vi "Source and Measure Current in DMM.vi"() -> ()   [LabVIEW 2021]
uses:
  <instrlib>/niDCPower/nidcpower.llb/niDCPower Source Mode.ctl
  <instrlib>/niDCPower/nidcpower.llb/niDCPower Wait For Event - Event.ctl
  <instrlib>/niDCPower/nidcpower.llb/niDCPower Output Function.ctl
  <instrlib>/niDMM/nidmm.llb/niDMM Function.ctl
  <instrlib>/niDMM/nidmm.llb/niDMM Configure Measurement Digits.vi
  <instrlib>/Agilent 3446X Series/Public/Data/Read (Single Point).vi
  <instrlib>/Agilent N6700 Series/Agilent N6700 Series.lvlib
  <instrlib>/Agilent 3446X Series/Agilent 3446X Series.lvlib
panel:
  in  "Agilent SMU":refnum<visa-resource-name>
  in  "Agilent SMU Channel":string="1"
  in  "Voltage Level":dbl=5.0 format="%^.3e"
  out "SMU Voltage Measurement":dbl format="%^.3e"
  in  "Current Limit":dbl=1.0 format="%^.3e"
  out "DMM Voltage Measurement":dbl
  in  "Manual Range":dbl=1.0
  in  "Agilent DMM":refnum<visa-resource-name>
  in  "Absolute Resolution":dbl=1e-06
  in  "Measurement Function":i32(ring)=10 items=["Continuity", "Current AC", "Current DC", "Diode", "Frequency", "Resistance 4-wire", "Period", "Resistance 2-wire", "Temperature", "Voltage AC", "Voltage DC", "Voltage DC Ratio", "Capacitance"]
  in  "Load DMM":refnum<k15>="Dev1"
  out "Current in DMM":dbl caption="Load SMU Current"
  in  "Resolution in Digits":dbl(ring)=5.5 items=["3 1/2"=3.5, "4 1/2"=4.5, "5 1/2"=5.5, "6 1/2"=6.5, "7 1/2"=7.5]
  in  "Range (Amps)":dbl=0.2 format="%.2p"
  in  "error in":errorcluster
  out "error out":errorcluster
  out "Voltage Measurement":dbl caption="Load SMU Voltage"
  out "Current Measurement":dbl caption="Load SMU Current"
  in  "Voltage Limit":dbl=2.0 format="%.5p"
  in  "Current Level":dbl=0.01 format="%.3p"
  in  "Load SMU Channel":string="0"
  in  "Load SMU":refnum<k15>="Dev1"
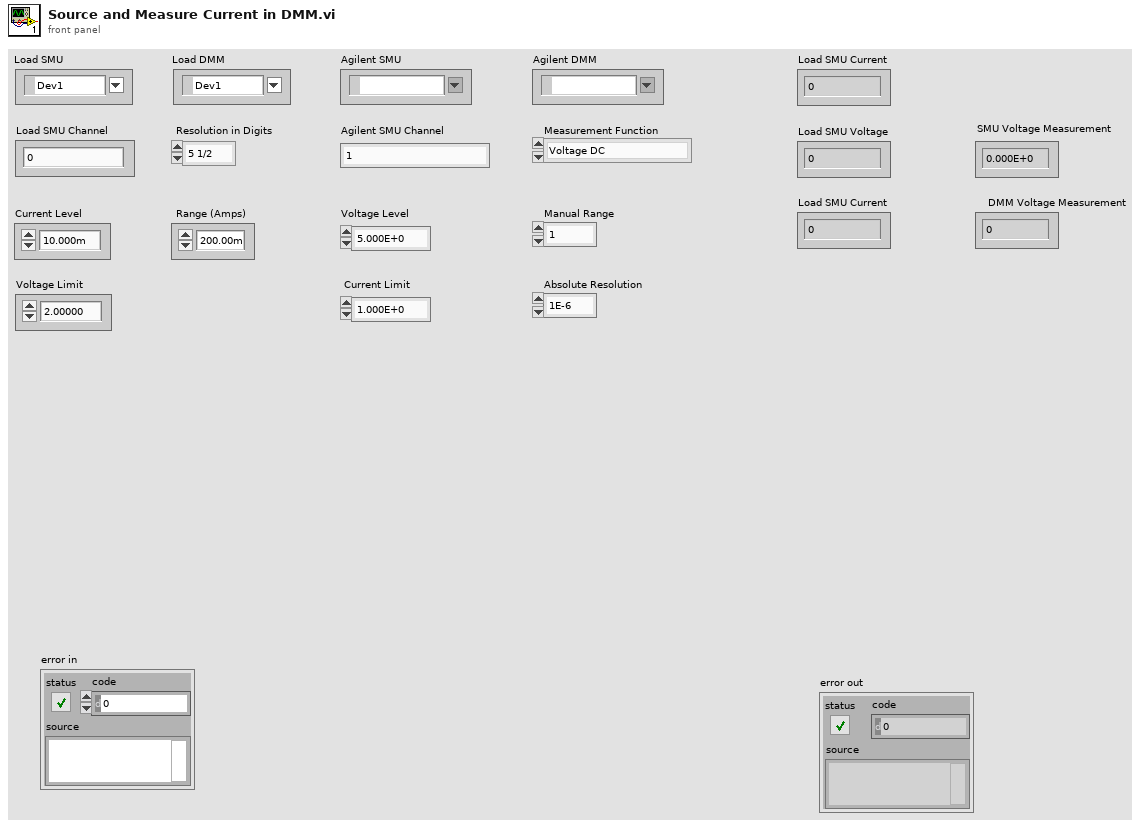
[diagram p1: front panel]
types:
  T1 = typedef "niDMM Function.ctl" = enum16{"DC Volts", "AC Volts", "DC Current", "AC Current", "2-wire Resistance", "4-wire Resistance", "Diode", "Frequency", "Period", "AC Volts DC Coupled", "Capacitance", "Inductance", "Temperature"}
  T2 = typedef "niDCPower Output Function.ctl" = i32
  T3 = typedef "niDCPower Wait For Event - Event.ctl" = i32
  T4 = typedef "niDCPower Source Mode.ctl" = i32
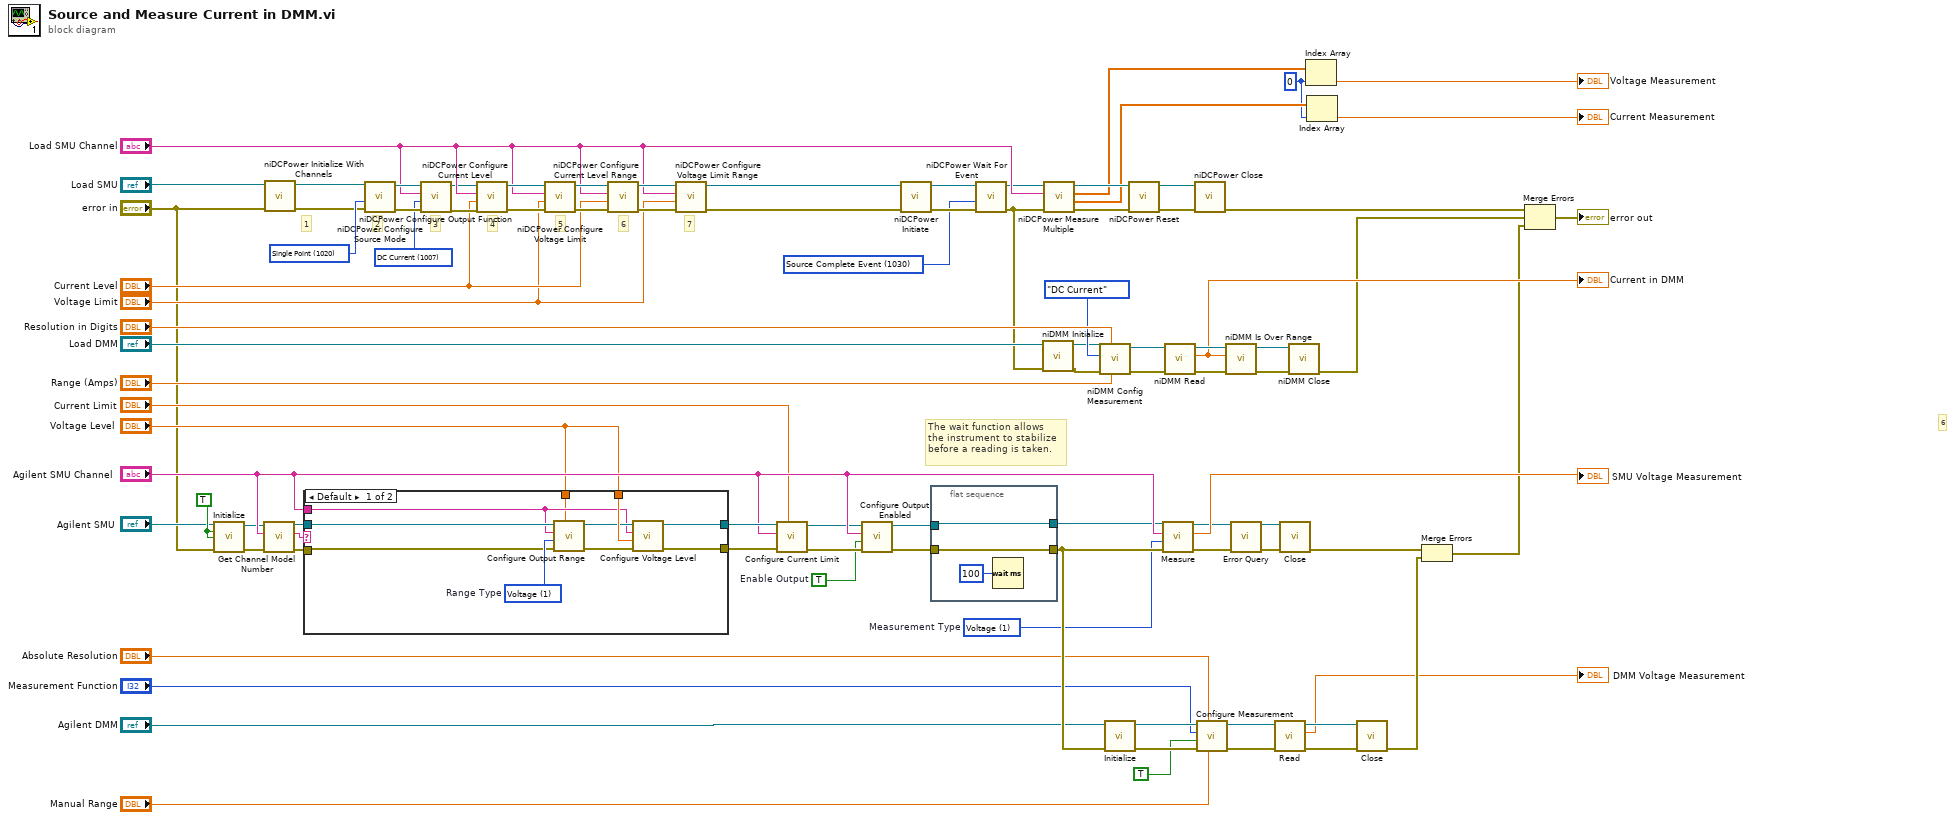
[diagram p0: block diagram]
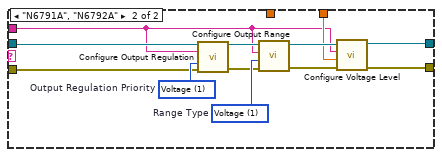
[diagram p2: hidden frame]
diagram:
  w14 = TRUE ("Reset? (T: Yes)")
  w13 = 1 items=["Voltage"=1, "Current"=0]  # Measurement Type
  w12 = TRUE  # Enable Output
  w67 = T2 1007 items=["DC Voltage"=1006, "DC Current"=1007, "Pulse Voltage"=1049, "Pulse Current"=1050] ("output function")
  w70 = T3 1030 items=["Source Complete Event"=1030, "Measure Complete Event"=1031, "Sequence Iteration Complete Event"=1032, "Sequence Engine Done Event"=1033] ("event")
  w79 = 0 ("index")
  w87 = T4 1020 items=["Single Point"=1020, "Sequence"=1021] ("source mode")
  # "The wait function allows \nthe instrument to stabilize\nbefore a reading is taken."
  # "6"
  # "7"
  # "6"
  # "2"
  # "3"
  # "5"
  # "4"
  # "1"
  n1 = call <instrlib>:"Initialize.vi"("VISA resource name"="Agilent SMU", "ID Query? (T: Yes)"=w14, "Reset? (T: Yes)"=w14, "error in (no error)"="error in") -> ("VISA resource name out"=w21:refnum<visa-resource-name>, "error out"=w22:errorcluster)  [unwired: 10 in]
  n2 = call <instrlib>:"Get Channel Model Number.vi"("error in (no error)"=w22, "Channel Name (1)"="Agilent SMU Channel", "VISA resource name"=w21) -> ("error out"=w24:errorcluster, "Model Number"=w25:string, "VISA resource name out"=w23:refnum<visa-resource-name>)  [unwired: 6 in]
  n3 = call <instrlib>:"niDCPower Initialize With Channels.vi"("error in (no error)"="error in", "resource name"="Load SMU") -> ("error out"=w52:errorcluster, "instrument handle out"=w53:refnum<k15>)  [unwired: 8 in]
  n4 = case shown="Default" w25 {
    tunnel: "Agilent SMU Channel" -> [w93 w104]
    tunnel: w23 -> [w100 w109]
    tunnel: w24 -> [w99 w108]
    tunnel: "Voltage Level" -> [w97 w105]
    tunnel: [w95 w102] -> w27
    tunnel: [w94 w103] -> w28
    tunnel: "Voltage Level" -> [w92 _]
    frame Default {
      w101 = 1 items=["Voltage"=1, "Current"=0]  # Range Type
      n5 = call <instrlib>:"Configure Output Range.vi"("Range (0.0)"=w92, "error in (no error)"=w99, "Range Type (1: Voltage)"=w101, "Channel Name (1)"=w93, "VISA resource name"=w100) -> ("error out"=w98:errorcluster, "VISA resource name out"=w96:refnum<visa-resource-name>)  [unwired: 5 in]
      n6 = call <instrlib>:"Configure Voltage Level.vi"("error in (no error)"=w98, "Level  (0.0 volts)"=w97, "Channel Name (1)"=w93, "VISA resource name"=w96) -> ("error out"=w95:errorcluster, "VISA resource name out"=w94:refnum<visa-resource-name>)  [unwired: 6 in]
    }
    frame "N6791A", "N6792A" {
      w110 = 1 items=["Voltage"=1, "Current"=0]  # Output Regulation Priority
      w113 = 1 items=["Voltage"=1, "Current"=0]  # Range Type
      n7 = call <instrlib>:"Configure Output Regulation.vi"("VISA resource name"=w109, "Channel Name (1)"=w104, "Output Regulation Priority (1: Voltage)"=w110, "error in (no error)"=w108) -> ("VISA resource name out"=w112:refnum<visa-resource-name>, "error out"=w111:errorcluster)  [unwired: 10 in]
      n8 = call <instrlib>:"Configure Output Range.vi"("error in (no error)"=w111, "Range Type (1: Voltage)"=w113, "Channel Name (1)"=w104, "VISA resource name"=w112) -> ("error out"=w106:errorcluster, "VISA resource name out"=w107:refnum<visa-resource-name>)  [unwired: 6 in]
      n9 = call <instrlib>:"Configure Voltage Level.vi"("error in (no error)"=w106, "Level  (0.0 volts)"=w105, "Channel Name (1)"=w104, "VISA resource name"=w107) -> ("error out"=w102:errorcluster, "VISA resource name out"=w103:refnum<visa-resource-name>)  [unwired: 6 in]
    }
  }
  n10 = call <instrlib>:"niDCPower Configure Source Mode.vi"("error in (no error)"=w52, "source mode"=w87, "instrument handle"=w53) -> ("error out"=w89:errorcluster, "instrument handle out"=w88:refnum<k15>)  [unwired: 7 out]
  n11 = call <instrlib>:"niDCPower Configure Output Function.vi"("error in (no error)"=w89, "output function"=w67, "channel name"="Load SMU Channel", "instrument handle"=w88) -> ("error out"=w69:errorcluster, "instrument handle out"=w68:refnum<k15>)  [unwired: 6 out]
  n12 = call <instrlib>:"niDCPower Configure Current Level.vi"("error in (no error)"=w69, "current level"="Current Level", "channel name"="Load SMU Channel", "instrument handle"=w68) -> ("error out"=w90:errorcluster, "instrument handle out"=w91:refnum<k15>)  [unwired: 6 out]
  n13 = call <instrlib>:"niDCPower Configure Voltage Limit.vi"("error in (no error)"=w90, "voltage limit"="Voltage Limit", "channel name"="Load SMU Channel", "instrument handle"=w91) -> ("error out"=w86:errorcluster, "instrument handle out"=w85:refnum<k15>)  [unwired: 6 out]
  n14 = call <instrlib>:"niDCPower Configure Current Level Range.vi"("error in (no error)"=w86, "current level range"="Current Level", "channel name"="Load SMU Channel", "instrument handle"=w85) -> ("error out"=w84:errorcluster, "instrument handle out"=w83:refnum<k15>)  [unwired: 6 out]
  n15 = call <instrlib>:"niDCPower Configure Voltage Limit Range.vi"("error in (no error)"=w84, "voltage limit range"="Voltage Limit", "channel name"="Load SMU Channel", "instrument handle"=w83) -> ("error out"=w75:errorcluster, "instrument handle out"=w76:refnum<k15>)  [unwired: 6 out]
  n16 = call <instrlib>:"Configure Current Limit.vi"("Limit (0.0 amps)"="Current Limit", "error in (no error)"=w27, "Channel Name (1)"="Agilent SMU Channel", "VISA resource name"=w28) -> ("error out"=w15:errorcluster, "VISA resource name out"=w16:refnum<visa-resource-name>)  [unwired: 6 in]
  n17 = call <instrlib>:"Configure Output Enabled.vi"("error in (no error)"=w15, "Enable Output (False)"=w12, "Channel Name (1)"="Agilent SMU Channel", "VISA resource name"=w16) -> ("error out"=w20:errorcluster, "VISA resource name out"=w18:refnum<visa-resource-name>)  [unwired: 6 in]
  n18 = call <instrlib>:"niDCPower Initiate.vi"("error in (no error)"=w75, "instrument handle"=w76) -> ("error out"=w71:errorcluster, "instrument handle out"=w73:refnum<k15>)  [unwired: 2 in, 6 out]
  n19 = flat-sequence {
    tunnel: w18 -> [w116]
    tunnel: [w116] -> w19
    tunnel: [w114] -> w42
    tunnel: w20 -> [w114]
    frame #0 {
      n20 = Wait (ms)(milliseconds to wait=u32 100) -> ()  [unwired: 1 out]
    }
  }
  n21 = call <instrlib>:"niDCPower Wait For Event.vi"("error in (no error)"=w71, "event"=w70, "instrument handle"=w73) -> ("error out"=w49:errorcluster, "instrument handle out"=w72:refnum<k15>)  [unwired: 1 in, 6 out]
  n22 = call <instrlib>:"niDMM Initialize.vi"("error in (no error)"=w49, "Instrument Descriptor"="Load DMM") -> ("error out"=w48:errorcluster, "instrument handle out"=w50:refnum<k15>)  [unwired: 8 in]
  n23 = call <instrlib>:"niDCPower Measure Multiple.vi"("error in (no error)"=w49, "channel name"="Load SMU Channel", "instrument handle"=w72) -> ("error out"=w57:errorcluster, "current measurements"=w80:dbl[], "voltage measurements"=w81:dbl[], "instrument handle out"=w82:refnum<k15>)  [unwired: 5 out]
  n24 = call-poly <instrlib>:"niDMM Config Measurement.vi"("Range"="Range (Amps)", "Resolution in Digits"="Resolution in Digits", "error in (no error)"=w48, "Function"=niDMM_Function."DC Current", "instrument handle"=w50) -> ("error out"=w65:errorcluster, "instrument handle out"=w64:refnum<k15>)  [unwired: 5 in]
  n25 = call <instrlib>:"Initialize.vi"("error in (no error)"=w42, "VISA resource name"="Agilent DMM") -> ("error out"=w39:errorcluster, "VISA resource name out"=w40:refnum<visa-resource-name>)  [unwired: 3 in, 5 out]
  n26 = call <instrlib>:"niDCPower Reset.vi"("error in (no error)"=w57, "instrument handle"=w82) -> ("error out"=w58:errorcluster, "instrument handle out"=w46:refnum<k15>)  [unwired: 2 in, 6 out]
  n27 = call <instrlib>:"Measure.vi"("error in (no error)"=w42, "Measurement Type (1: Voltage)"=w13, "Channel Name (1)"="Agilent SMU Channel", "VISA resource name"=w19) -> ("error out"=w6:errorcluster, "Measurement"=→"SMU Voltage Measurement":dbl, "VISA resource name out"=w9:refnum<visa-resource-name>)  [unwired: 5 in]
  n28 = call <instrlib>:"niDMM Read.vi"("error in (no error)"=w65, "instrument handle"=w64) -> ("error out"=w62:errorcluster, "Measurement"=w55:dbl, "instrument handle out"=w63:refnum<k15>)  [unwired: 7 in]
  "Current in DMM" <- w55
  n29 = call <instrlib>:"niDCPower Close.vi"("error in (no error)"=w58, "instrument handle"=w46) -> ("error out"=w47:errorcluster)  [unwired: 9 in]
  n30 = call <instrlib>:"Configure Measurement.vi"("Manual Range (1)"="Manual Range", "Absolute Resolution (1E-6)"="Absolute Resolution", "error in (no error)"=w39, "Auto Range (T: Enable)"=TRUE, "Measurement Function (10: Voltage DC)"="Measurement Function", "VISA resource name"=w40) -> ("error out"=w35:errorcluster, "VISA resource name out"=w36:refnum<visa-resource-name>)  [unwired: 4 out]
  n31 = call <instrlib>:"niDMM Is Over Range.vi"("error in (no error)"=w62, "Measurement"=w55, "instrument handle"=w63) -> ("error out"=w61:errorcluster, "instrument handle out"=w44:refnum<k15>)  [unwired: 6 in, 1 out]
  n32 = call <instrlib>:"Error Query.vi"("VISA resource name"=w9, "error in (no error)"=w6) -> ("VISA resource name out"=w8:refnum<visa-resource-name>, "error out"=w7:errorcluster)  [unwired: 10 in, 2 out]
  n33 = call-poly <instrlib>:"Read.vi"("error in (no error)"=w35, "VISA resource name"=w36) -> ("error out"=w38:errorcluster, "Measurement"=→"DMM Voltage Measurement":dbl, "VISA resource name out"=w37:refnum<visa-resource-name>)  [unwired: 7 out]
  n34 = call <instrlib>:"Close.vi"("VISA resource name"=w8, "error in (no error)"=w7) -> ("error out"=w41:errorcluster)  [unwired: 13 in]
  n35 = call <instrlib>:"niDMM Close.vi"("error in (no error)"=w61, "instrument handle"=w44) -> ("error out"=w45:errorcluster)  [unwired: 9 in]
  n36 = Index Array(array=w81, index=w79) -> (element=→"Voltage Measurement":dbl)
  n37 = Index Array(array=w80, index=w79) -> (element=→"Current Measurement":dbl)
  n38 = call <instrlib>:"Close.vi"("error in (no error)"=w38, "VISA resource name"=w37) -> ("error out"=w43:errorcluster)  [unwired: 9 out]
  n39 = Merge Errors(w41, w43) -> (w5:errorcluster)
  n40 = Merge Errors(w47, w45, w5) -> (→"error out":errorcluster)
